vi "Launch Wizard.vi"(8 "error in (no error)":errorcluster, 10 "Controller in":refnum<class "Controller.lvclass">, 11 "UI Wizard in":refnum<class "UI Wizard.lvclass">) -> (0 "error out":errorcluster, 3 "Caller-To-Actor Enqueuer":refnum<class "Message Enqueuer.lvclass">)   [LabVIEW 2013, in "SET Project Editor.lvlib" / "UI Wizard.lvclass"]
uses:
  UI Wizard.lvclass
  <vilib>/ActorFramework/Message Enqueuer/Message Enqueuer.lvclass
  Controller/Controller.lvclass
  <vilib>/ActorFramework/Actor/Actor.lvclass/Actor.ctl
  <vilib>/ActorFramework/Message Enqueuer/Message Enqueuer.lvclass/Message Enqueuer.ctl
  UI Wizard.lvclass/UI Wizard.ctl
  <vilib>/ActorFramework/Message Enqueuer/Init from Existing Queue.vi
  <vilib>/ActorFramework/Actor/Actor.lvclass
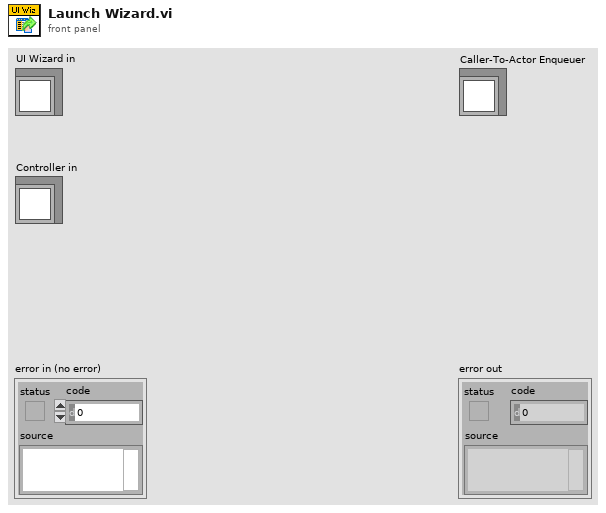
[diagram p1: front panel]
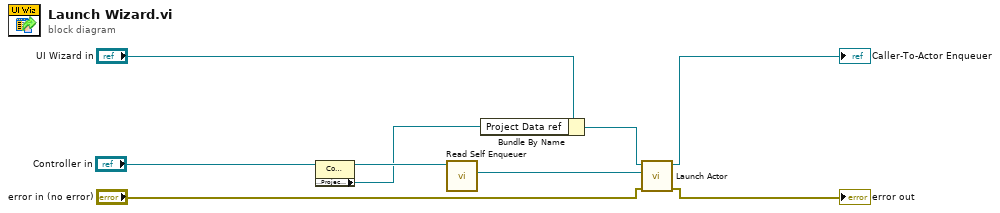
[diagram p0: block diagram]
diagram:
  n1 = property class="Controller.lvclass"(reference="Controller in") -> (reference out=w5:refnum<class "Controller.lvclass">, "Properties:Project Data ref"=w1:refnum<data-value>)  [unwired: 1 in, 1 out]
  n2 = call <vilib>:"Read Self Enqueuer.vi"("Actor"=w5) -> ("Self Enqueuer"=w7:refnum<class "Message Enqueuer.lvclass">)  [unwired: 10 in]
  n3 = Bundle By Name(cluster="UI Wizard in", "Project Data ref"=w1) -> (w6:refnum<class "UI Wizard.lvclass">)
  n4 = call <vilib>:"Launch Actor.vi"("error in (no error)"="error in (no error)", "Actor-to-Caller Enqueuer"=w7, "Actor"=w6) -> ("error out"=→"error out":errorcluster, "Caller-To-Actor Enqueuer"=→"Caller-To-Actor Enqueuer":refnum<class "Message Enqueuer.lvclass">)  [unwired: 7 in]
